vi "Simple Reader.vi"(8 "error in (no error)":errorcluster, 11 "Keithley Driver in":refnum<class "Keithley Driver.lvclass">) -> (0 "error out":errorcluster, 2 "Signals":dbl[](array[numeric]), 3 "Keithley Driver out":refnum<class "Keithley Driver.lvclass">)   [LabVIEW 2016, in "Keithley Driver.lvclass"]
uses:
  Keithley Driver.lvclass
  C:/github/NHMFL_Core/Libraries/Instruments/VISA Instrument/VISA Instrument.lvclass
  VISA Instrument/VISA Instrument.lvclass/VISA Instrument.ctl
  VISA Instrument/Read VISA resource.vi
  VISA Instrument/Write VISA resource.vi
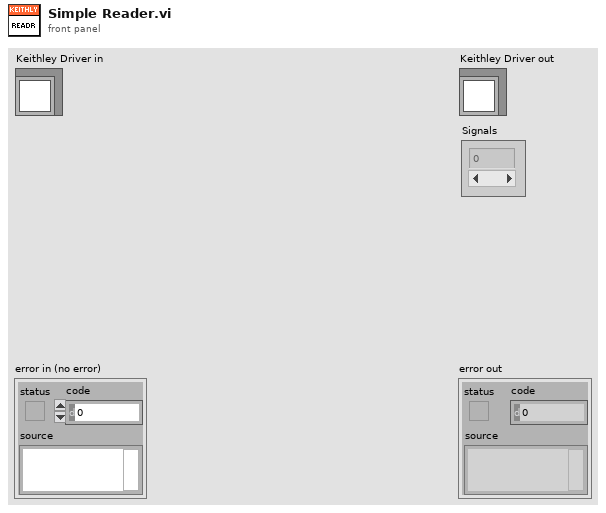
[diagram p1: front panel]
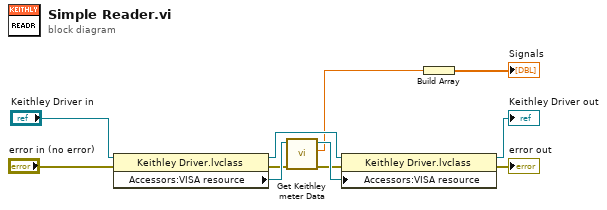
[diagram p0: block diagram]
diagram:
  n1 = property class="Keithley Driver.lvclass"(reference="Keithley Driver in", error in="error in (no error)") -> (reference out=w11:refnum<class "Keithley Driver.lvclass">, error out=w2:errorcluster, "Accessors:VISA resource"=w6:refnum<visa-resource-name>)
  n2 = call "Get Keithley meter Data.vi"("error in (no error)"=w2, "VISA Resource Name"=w6) -> ("error out"=w1:errorcluster, "Data"=w4:dbl, "VISA Resource Name Out"=w5:refnum<visa-resource-name>)  [unwired: 7 in]
  n3 = property class="Keithley Driver.lvclass"(reference=w11, error in=w1, "Accessors:VISA resource"=w5) -> (reference out=→"Keithley Driver out":refnum<class "Keithley Driver.lvclass">, error out=→"error out":errorcluster)
  n4 = Build Array(w4) -> (→"Signals":dbl[])
